vi "Pin Map XML Strings Global.vi"() -> ()   [LabVIEW 2020, in "MeasurementServerTests.lvlib"]
uses:
  MeasurementServerTests.lvlib
panel:
  in  "1Fgen1Pin1Site":string="<?xml version=\"1.0\" encoding=\"utf-8\"?>\n<PinMap xmlns=\"http://www.ni.com/TestStand/SemiconductorModule/PinMap.xsd\" xmlns:xsi=\"http://www.w3.org/2001/XMLSchema-instance\" schemaVersion=\"1.1\">\n\t<Instruments>\n\t\t<NIFGenInstrument name=\"FGEN1\" numberOfChannels=\"1\" />\n\t</Instruments>\n\t<Pins>\n\t\t<DUTPin name=\"Pin1\" />\n\t</Pins>\n\t<Sites>\n\t\t<Site siteNumber=\"0\" />\n\t</Sites>\n\t<Connections>\n\t\t<Connection pin=\"Pin1\" siteNumber=\"0\" instrument=\"FGEN1\" channel=\"0\" />\n\t</Connections>\n</PinMap>"
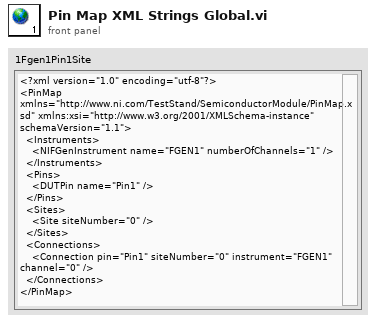
[diagram p1: front panel]
diagram:
